vi "add_JointCommand.vi"(8 "Mode":T1=1 items=["Position"=1, "Velocity"=2, "Effort"=3], 9 "names":string[](array[string]), 10 "command":dbl[](array[numeric]), 11 "msg in":string) -> (3 "msg out":string)   [LabVIEW 2010]
uses:
  std_msgs/subs/i32Scalar.vi
  std_msgs/subs/stringArray.vi
  std_msgs/subs/float64Array.vi
  Code/SubVIs/JointMode.ctl
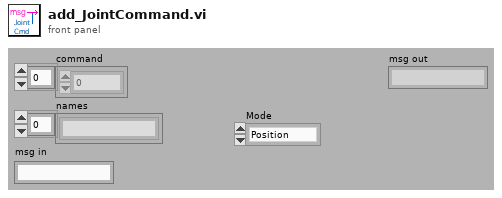
[diagram p1: front panel]
types:
  T1 = typedef "JointMode.ctl" = u8
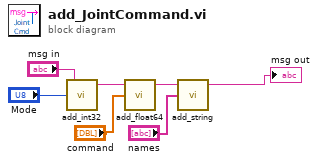
[diagram p0: block diagram]
diagram:
  n1 = call-poly "add_int32.vi"("Numeric"="Mode", "msg in"="msg in") -> ("msg out"=w7:string)  [unwired: 3 in]
  n2 = call-poly "add_float64.vi"("Array"="command", "msg in"=w7) -> ("msg out"=w6:string)  [unwired: 3 in]
  n3 = call-poly "add_string.vi"("Array"="names", "msg in"=w6) -> ("msg out"=→"msg out":string)  [unwired: 3 in]
